vi "Prepare messages based on command.vi"(8 "NoMessges":i32[](array[numeric]), 9 "DATA[X]":u8[](array[numeric]), 10 "Tx und Rx":T2(array[cluster]), 11 "Commands":T3) -> (2 "Expected messages":T1[](array[typedef]), 3 "Tx":T2(array[cluster]))   [LabVIEW 2025]
uses:
  Commands.ctl
  Expected messages.ctl
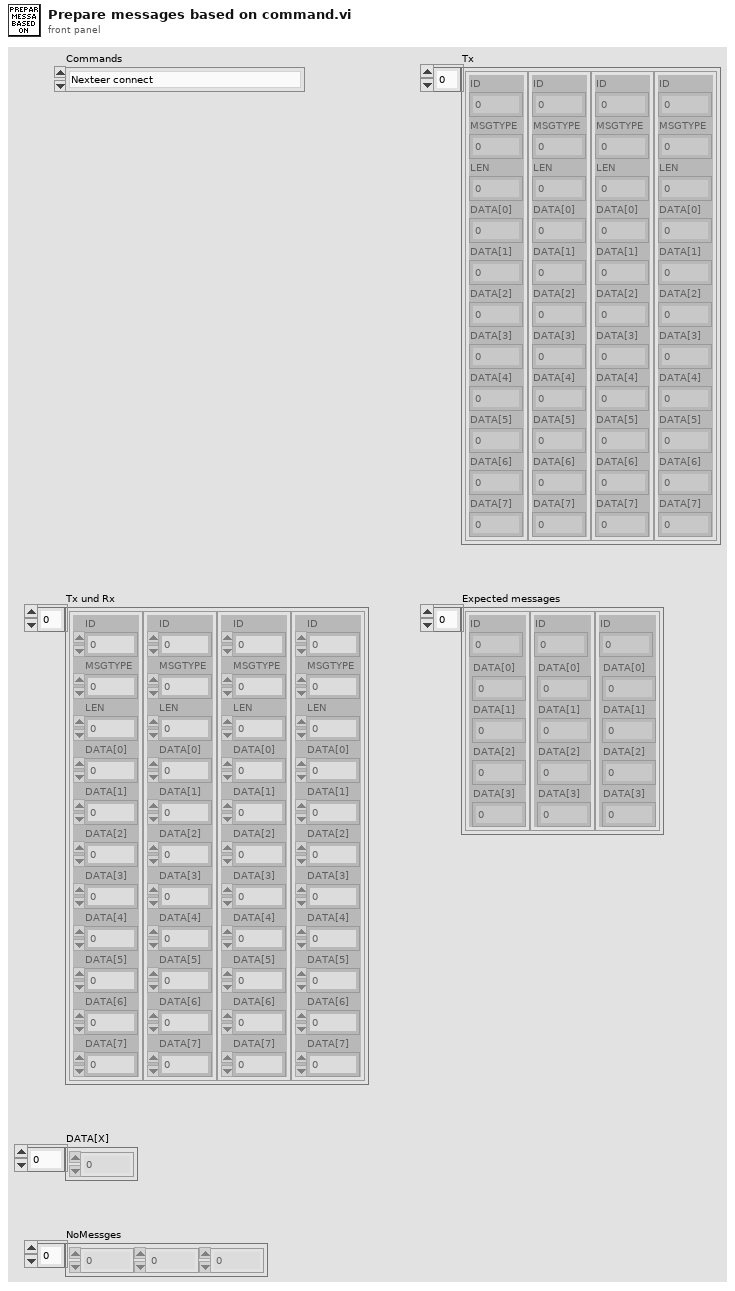
[diagram p1: front panel]
types:
  T1 = typedef "Expected messages.ctl" = cluster{"DATA[0]":u8, "DATA[1]":u8, "DATA[2]":u8, "DATA[3]":u8, "ID":u32}
  T2 = cluster{"ID":u32, "MSGTYPE":u8, "LEN":u8, "DATA[0]":u8, "DATA[1]":u8, "DATA[2]":u8, "DATA[3]":u8, "DATA[4]":u8, "DATA[5]":u8, "DATA[6]":u8, "DATA[7]":u8}[]
  T3 = typedef "Commands.ctl" = enum16{"Nexteer connect", "Write Polarity", "Write BEMF", "Write Torque Scale Sensors T1", "Write Torque Scale Sensors T2", "Trim HW Torque Sensors T1", "Trim HW Torque Sensors T2", "Read HW Torque Trim Performed Sensors T1", "Read HW Torque Trim Performed Sensors T2", "Write EOL Offset values to defaults", "Write EOL Gain values to defaults", "Write Serial Number", "Write Hardware Part Number", "Write EPS Serial Number", "Read MEC Counter", "MCU Reset", "Read System State", "Read First Motor Position", "Manufacturing Diagnostic Defeat", "Perform Current Offset ", "Current Offset Status", "Enable Engine Run", "Perform Current Gain ", "Current Gain Status", "Disable Torque Ramp Down ", "Disable Engine Run", "Set Vehicle Speed Override", "Read Offset Values Using FD F5", "Read Gain Values Using FD F4", "Clear Nexteer NTCs", "Read Second Motor Position", "Read ECU Software ID", "Read Internal Software Version", "Read Bootloader ID", "Read Bootloader Software Version", "Read Calibration Release 0", "Read Calibration Release 1", "Read Calibration Release 2", "Read Temperature  ", "Battery Voltage  ", "Read Motor Angle 0", "Read Motor Angle 1 ", "Set Motor Torque Command ", "Read Motor Current   ", "Stop Motor Torque Command", "Read NTCs", "Read Serial Number", "Read HW Part Number", "Read Polarity", "Set NVM Access Defeat", "Read Software Release", "Read Software Build Date", "Write Single Inverter Hardware value", "Write Dual Inverter Hardware value", "Read Single Inverter HW Value", "Read Dual Inverter HW Value", "Write MEC Counter FE", "Write MEC Counter FF", "Read BEMF", "Read Torque 1 FDB6", "Read Torque 2 FDB7", "Read Torque Trim 1 FDB4", "Read Torque Trim 2 FDB5", "Write Torque Trim 1 FDB4", "Write Torque Trim 2 FDB5", "XCP connect", "Read HW Torque T1", "Read HW Torque T2", "Read Motor Speed "}
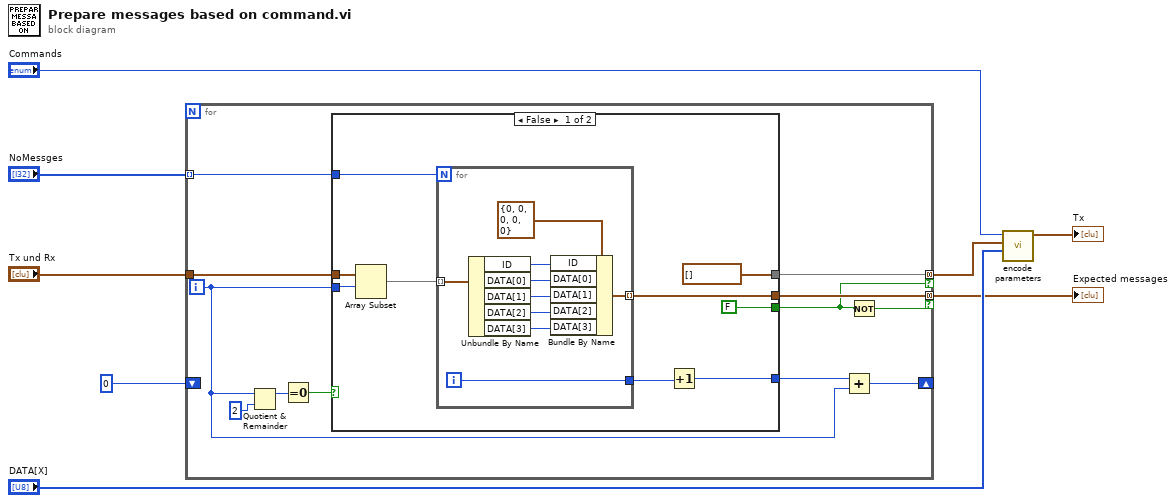
[diagram p0: block diagram]
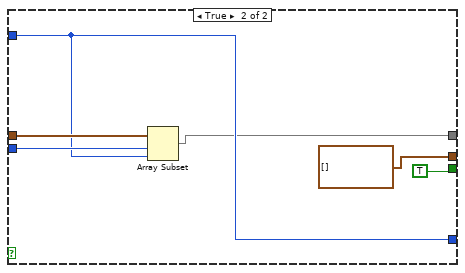
[diagram p2: hidden frame]
diagram:
  n1 = for {
    tunnel: "NoMessges" -> [w17] mode=indexing
    tunnel: "Tx und Rx" -> [w16]
    tunnel: [w13] -> w5 mode=concatenating if=w11
    shift-right: [w15] -> _
    shift-left: 0 -> [_]
    tunnel: [w14] -> w2 mode=concatenating if=w12
    i -> [w10]
    n2 = Quotient & Remainder(x=w10, y=2) -> (x-y*floor(x/y)=w19:i32)  [unwired: 1 out]
    n3 = Equal To 0?(x=w19) -> (x = 0?=w18:bool)
    n4 = case shown="False" w18 {
      tunnel: w17 -> [w29 w40]
      tunnel: w16 -> [w28 w42]
      tunnel: [T2 [] w39] -> w13
      tunnel: [w26 T1[] []] -> w14
      tunnel: [FALSE TRUE] -> w11
      tunnel: [w22 w40] -> w9
      tunnel: w10 -> [w21 w41]
      frame False {
        n5 = Array Subset(array=w28, index=w21) -> (w27:T2)  [unwired: 1 in]
        n6 = for {
          N: w29 -> [_]
          tunnel: w27 -> [w37] mode=indexing
          tunnel: [w36] -> w23
          tunnel: [w31] -> w26 mode=indexing
          i -> [w36]
          n7 = Unbundle By Name(w37) -> ("ID"=w30:u32, "DATA[0]"=w35:u8, "DATA[1]"=w34:u8, "DATA[2]"=w33:u8, "DATA[3]"=w32:u8)
          n8 = Bundle By Name(cluster=T1 {"DATA[0]"=0, "DATA[1]"=0, "DATA[2]"=0, "DATA[3]"=0, "ID"=0} ("Expected responses"), "ID"=w30, "DATA[0]"=w35, "DATA[1]"=w34, "DATA[2]"=w33, "DATA[3]"=w32) -> (w31:T1)
        }
        n9 = Increment(x=w23) -> (x+1=w22:i32)
      }
      frame True {
        n10 = Array Subset(array=w42, index=w41, length=w40) -> (w39:T2)
      }
    }
    n11 = Add(x=w9, y=w10) -> (x+y=w15:i32)
    n12 = Not(x=w11) -> (.not. x?=w12:bool)
  }
  "Expected messages" <- w2
  n13 = call "encode parameters.vi"("DATA[X]"="DATA[X]", "Tx in"=w5, "Commands"="Commands") -> ("Tx out"=→"Tx":T2)  [unwired: 8 in]
